vi "Hex to Dec.vi"(8 "Error In":errorcluster, 10 "Max Value":dbl, 11 "Hexadecimal Value":u8) -> (0 "Error Out":errorcluster, 3 "Decimal Value":dbl)   [LabVIEW 2023, in "Decoder.lvlib"]
doc: "Transfer hexadecimalvalue to decimal"
uses:
  Decoder.lvlib
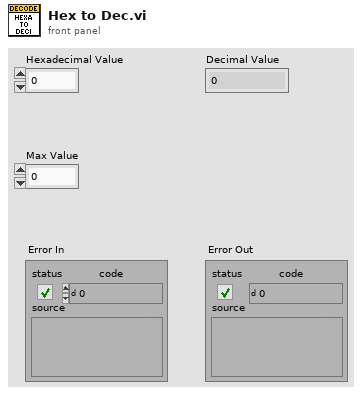
[diagram p1: front panel]
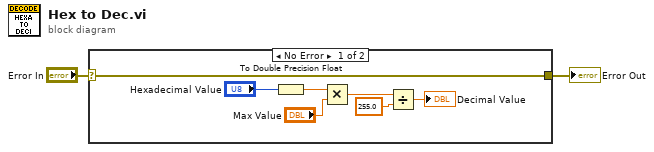
[diagram p0: block diagram]
diagram:
  n1 = case shown="No Error" "Error In" {
    selector: "Error In" -> [w3 w10]
    tunnel: [w3 w10] -> w1
    frame No Error {
      n2 = To Double Precision Float(number="Hexadecimal Value") -> (double precision float=w9:dbl)
      n3 = Multiply(x=w9, y="Max Value") -> (x*y=w8:dbl)
      n4 = Divide(x=w8, y=255.0) -> (x/y=→"Decimal Value":dbl)
    }
    frame Error {
    }
  }
  "Error Out" <- w1
